vi "check for errors.vi"(8 "error in":errorcluster, 11 "function return":i32=-1) -> (0 "error out":errorcluster)   [LabVIEW 2013, in "lvnano.lvlib"]
uses:
  lvnano.lvlib
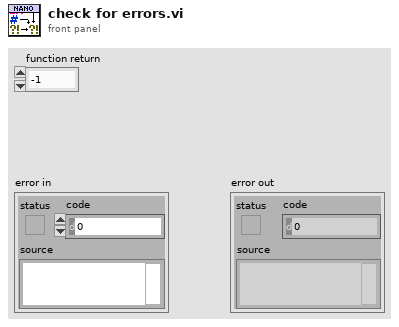
[diagram p1: front panel]
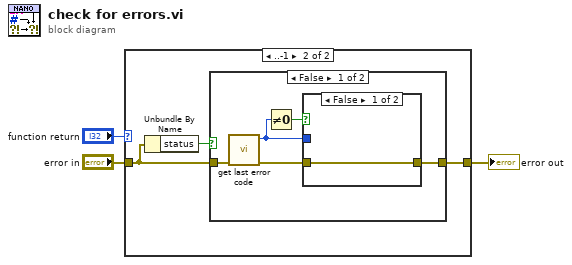
[diagram p0: block diagram]
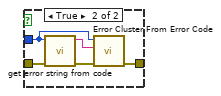
[diagram p3: hidden frame]
diagram:
  n1 = case shown="..-1" "function return" {
    tunnel: [w4 w7] -> w2
    tunnel: "error in" -> [w4 w6]
    frame 0.. {
    }
    frame ..-1 {
      n2 = Unbundle By Name(w6) -> ("status"=w5:bool)
      n3 = case shown="False" w5 {
        tunnel: [w11 w19] -> w7
        tunnel: w6 -> [w9 w19]
        frame False {
          n4 = call "get last error code.vi"("error in (no error)"=w9) -> ("error out"=w8:errorcluster, "function return"=w10:i32)  [unwired: 9 in]
          n5 = Not Equal To 0?(x=w10) -> (x != 0?=w12:bool)
          n6 = case shown="False" w12 {
            tunnel: w8 -> [w13 w17]
            tunnel: w10 -> [_ w15]
            tunnel: [w13 w18] -> w11
            frame False {
            }
            frame True {
              n7 = call "get error string from code.vi"("error in (no error)"=w17, "errnum"=w15) -> ("error out"=w16:errorcluster, "function return"=w14:string)  [unwired: 8 in]
              n8 = call <vilib>:"Error Cluster From Error Code.vi"("error in (no error)"=w16, "error message (\"\")"=w14, "error code (0)"=w15) -> ("error out"=w18:errorcluster)  [unwired: 6 in]
            }
          }
        }
        frame True {
        }
      }
    }
  }
  "error out" <- w2
